vi "CreateComponentFolder.vi"(8 "error in (no error)":errorcluster, 10 "Component Idx":i32, 11 "Current Path":path) -> (0 "error out":errorcluster, 3 "created path":path)   [LabVIEW 2017]
doc: "Creates the folder for component and diagram"
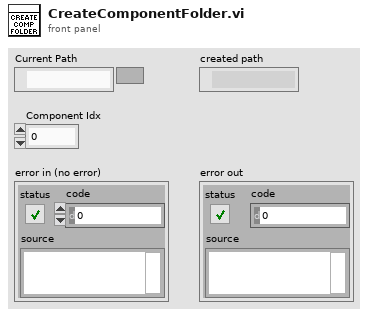
[diagram p1: front panel]
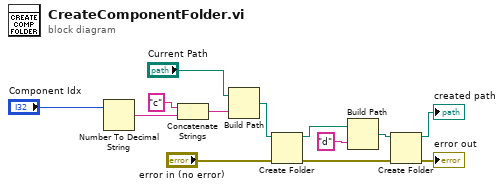
[diagram p0: block diagram]
diagram:
  n1 = Number To Decimal String(number="Component Idx") -> (decimal integer string=w11:string)  [unwired: 1 in]
  n2 = Concatenate Strings("c" ("string"), w11) -> (w5:string)
  n3 = Build Path(base path="Current Path", name or relative path=w5) -> (appended path=w4:path)
  n4 = Create Folder(path (use dialog)=w4, error in="error in (no error)") -> (created path=w2:path, error out=w7:errorcluster)  [unwired: 1 in, 1 out]
  n5 = Build Path(base path=w2, name or relative path="d" ("string")) -> (appended path=w1:path)
  n6 = Create Folder(path (use dialog)=w1, error in=w7) -> (created path=→"created path":path, error out=→"error out":errorcluster)  [unwired: 1 in, 1 out]
